vi "RSZVB Set Source Power Calibration Convergence Factor.vi"(8 "error in (no error)":errorcluster {"code" format="%.0x"}, 10 "Convergence Factor (0)":dbl=1.0 format="%^.3e", 11 "VISA session":refnum<visa-resource-name>) -> (0 "error out":errorcluster {"code" format="%.0x"}, 3 "dup VISA session":refnum<visa-resource-name>)   [LabVIEW 2011]
doc: "Specifies the convergence factor for a source power calibration. \n\nRemote-control command(s):\nSOURce<Ch>:POWer<Pt>:CORRection:COLLect:CFACtor"
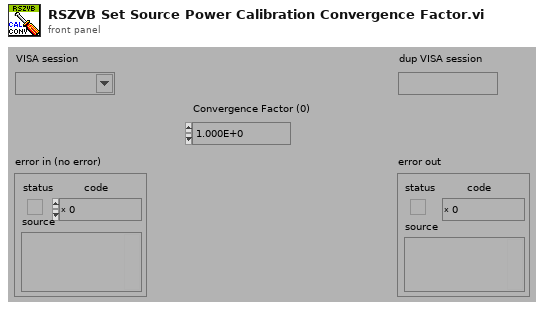
[diagram p1: front panel]
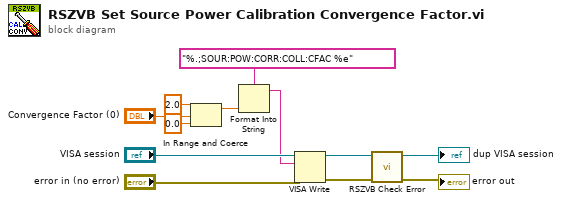
[diagram p0: block diagram]
diagram:
  n1 = In Range and Coerce(upper limit=2.0, x="Convergence Factor (0)", lower limit=0.0) -> (coerced(x)=w11:dbl)  [unwired: 1 out]
  n2 = Format Into String(format string="%.;SOUR:POW:CORR:COLL:CFAC %e", w11) -> (resulting string=w5:string)  [unwired: 2 in, 1 out]
  n3 = VISA Write(VISA resource name="VISA session", write buffer=w5, error in (no error)="error in (no error)") -> (VISA resource name out=w3:refnum<visa-resource-name>, error out=w4:errorcluster)  [unwired: 1 out]
  n4 = call "RSZVB Check Error.vi"("error in (no error)"=w4, "VISA session"=w3) -> ("error out"=→"error out":errorcluster, "dup VISA session"=→"dup VISA session":refnum<visa-resource-name>)  [unwired: 8 in]
